vi "TP Information.vi"(10 "TP information in":string[](array[string]), 11 "base path":path) -> (2 "TP Information out":string[](array[string]))   [LabVIEW 2018]
uses:
  Global.vi
panel:
  out "布尔":bool
  in  "Bar":bool
  in  "过程停止按钮":bool
  in  "HW Ch Number":string caption="硬体配置通道数"
  in  "Board COL":string caption="连板方式(列)"
  in  "Board ROW":string caption="连板方式(行)"
  in  "确定":bool
  in  "浏览":bool
  in  "hwfile":string caption="配置文件"
  in  "备注":string
  in  "author":string caption="用户："
  in  "Modulename":string caption="机种名称"
  # "X"
  # "="
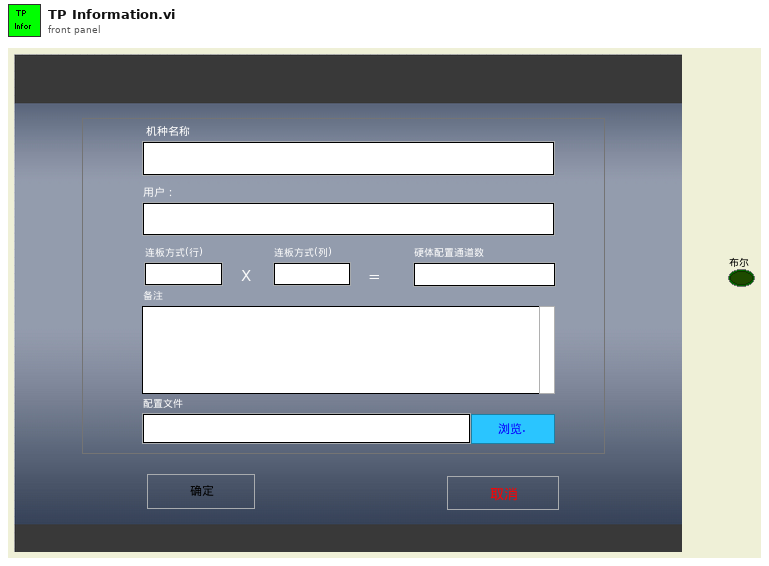
[diagram p1: front panel]
types:
  T1 = typedef "Window Refnum.ctl" = refnum<k1>
  T2 = typedef "Window Rectangle.ctl" = cluster{"left":i16, "top":i16, "right":i16, "bottom":i16}
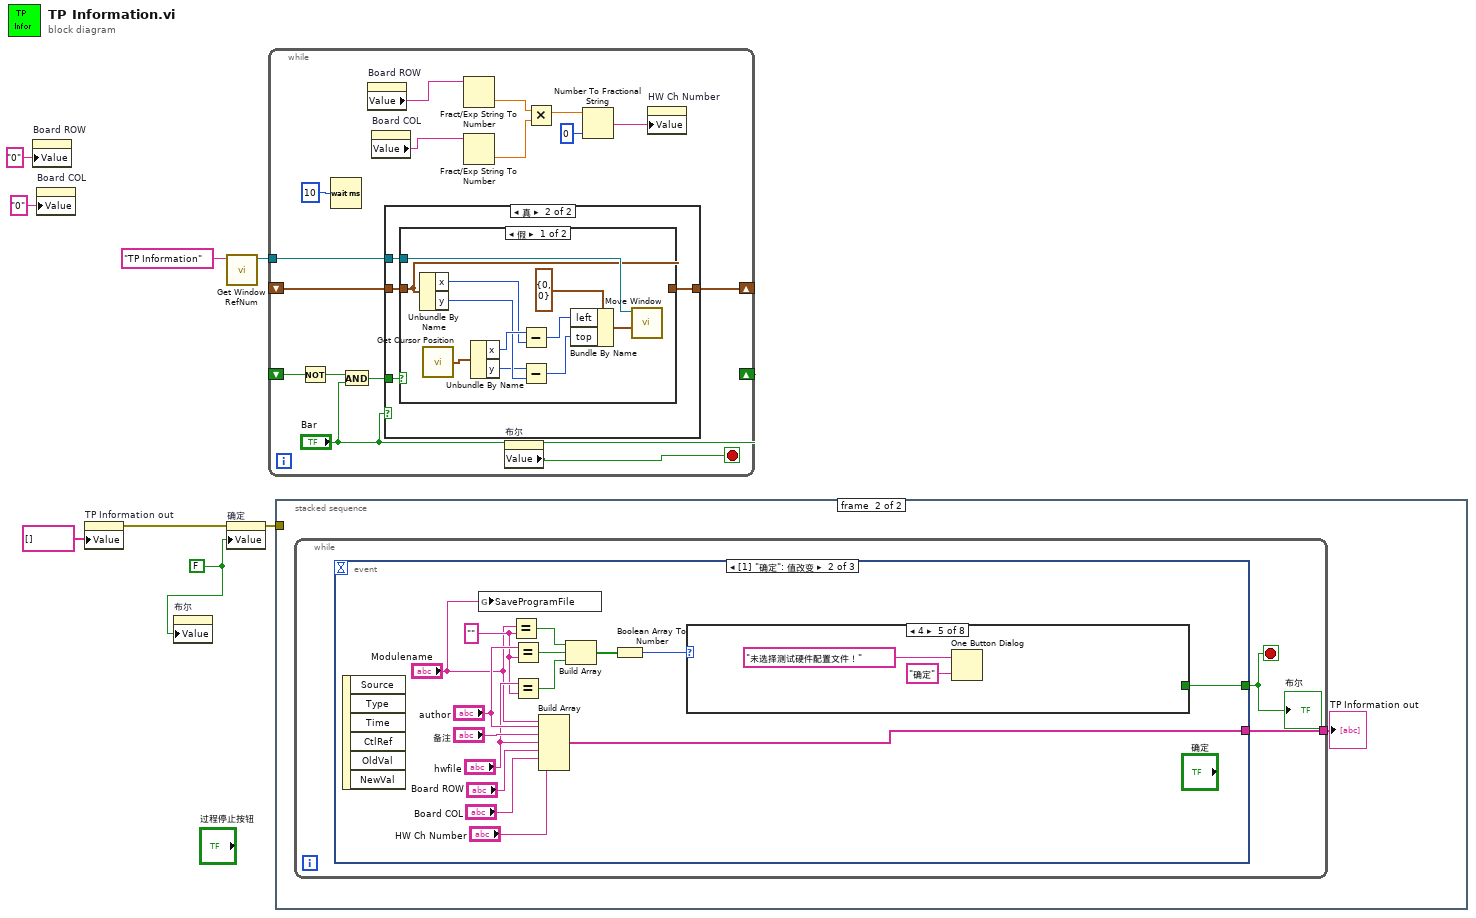
[diagram p0: block diagram]
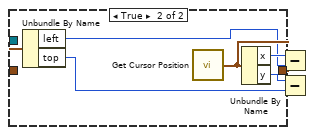
[diagram p3: hidden frame]
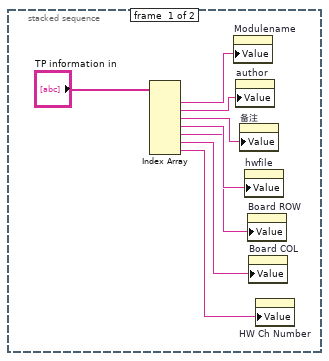
[diagram p4: hidden frame]
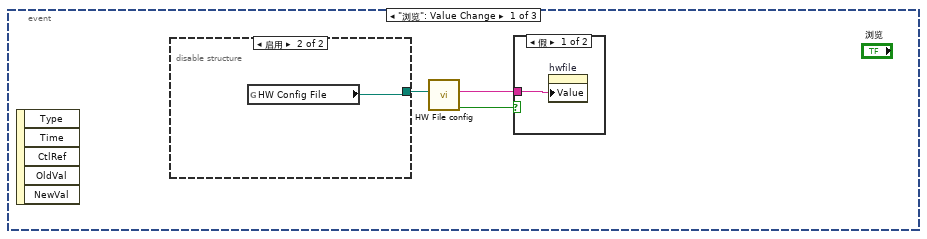
[diagram p5: hidden frame]
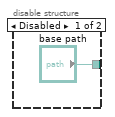
[diagram p6: hidden frame]
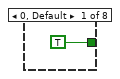
[diagram p8: hidden frame]
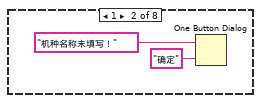
[diagram p9: hidden frame]
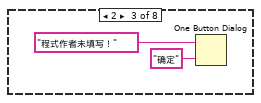
[diagram p10: hidden frame]
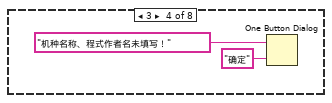
[diagram p11: hidden frame]
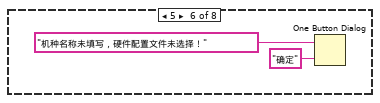
[diagram p12: hidden frame]
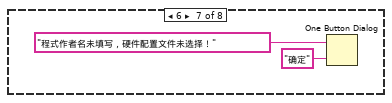
[diagram p13: hidden frame]
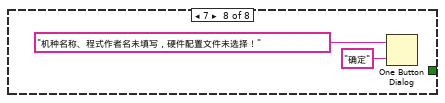
[diagram p14: hidden frame]
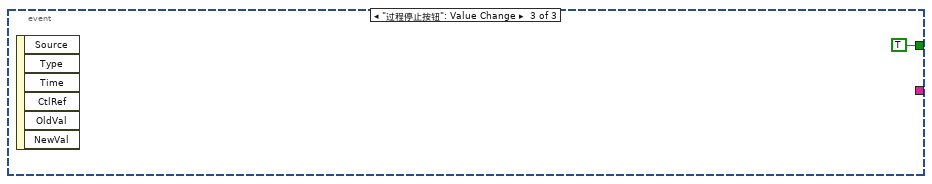
[diagram p15: hidden frame]
diagram:
  w3 = FALSE
  n1 = property on="Board ROW" class="Str"("Value"="0" ("Board ROW")) -> ()  [unwired: 2 in, 2 out]
  n2 = property on="Board COL" class="Str"("Value"="0" ("Board COL")) -> ()  [unwired: 2 in, 2 out]
  n3 = property on="TP Information out" class="Arr (严格)"("Value"=string[] []) -> (error out=w7:errorcluster)  [unwired: 2 in, 1 out]
  n4 = property on="布尔" class="Bool (严格)"("Value"=w3) -> ()  [unwired: 2 in, 2 out]
  n5 = call "Get Window RefNum.vi"("window name (\"\")"="TP Information" ("window name (\"\")")) -> ("window refnum (NaWR)"=w4:T1)  [unwired: 1 in, 7 out]
  n6 = property on="确定" class="Bool"(error in=w7, "Value"=w3) -> (error out=w8:errorcluster)  [unwired: 1 in, 1 out]
  n7 = while {
    shift-left: _ -> [w18]
    shift-right: [w19] -> _
    shift-left: _ -> [w22]
    shift-right: ["Bar"] -> _
    tunnel: w4 -> [w23]
    stop <- w16 stop-if-true
    n8 = Not(x=w22) -> (.not. x?=w21:bool)
    n9 = Wait (ms)(milliseconds to wait=u32 10) -> ()  [unwired: 1 out]
    n10 = And(x=w21, y="Bar") -> (x .and. y?=w17:bool)
    n11 = property on="Board ROW" class="Str"() -> ("Value"=w15:string)  [unwired: 2 in, 2 out]
    n12 = property on="Board COL" class="Str"() -> ("Value"=w14:string)  [unwired: 2 in, 2 out]
    n13 = case shown="真" "Bar" {
      tunnel: w23 -> [_ w29]
      tunnel: [w25 w28] -> w19
      tunnel: w18 -> [w25 w26]
      tunnel: w17 -> [_ w27]
      frame False {
      }
      frame True {
        n14 = case shown="假" w27 {
          tunnel: w29 -> [w35 w51]
          tunnel: [w30 w41] -> w28
          tunnel: w26 -> [w30 _]
          frame False {
            n15 = Unbundle By Name(w30) -> ("x"=w38:i16, "y"=w37:i16)
            n16 = call "Get Cursor Position.vi"() -> ("cursor position"=w40:cluster{"x":i16, "y":i16})
            n17 = Unbundle By Name(w40) -> ("x"=w39:i16, "y"=w36:i16)
            n18 = Subtract(x=w39, y=w38) -> (x-y=w32:i16)
            n19 = Subtract(x=w36, y=w37) -> (x-y=w33:i16)
            n20 = Bundle By Name(cluster=cluster{"left":i16, "top":i16} {"left"=0, "top"=0} ("new position (0,0)"), "left"=w32, "top"=w33) -> (w31:cluster{"left":i16, "top":i16})
            n21 = call "Move Window.vi"("new position (0,0)"=w31, "window refnum (NaWR)"=w35) -> ()  [unwired: 2 in, 4 out]
          }
          frame True {
            n22 = call "Get Window Rectangle.vi"("window refnum (NaWR)"=w51) -> ("window rect"=w50:T2)  [unwired: 1 in, 5 out]
            n23 = call "Extract Window Origin.vi"("window rect"=w50) -> ("window origin"=w49:cluster{"left":i16, "top":i16})  [unwired: 1 out]
            n24 = Unbundle By Name(w49) -> ("left"=w46:i16, "top"=w45:i16)
            n25 = call "Get Cursor Position.vi"() -> ("cursor position"=w48:cluster{"x":i16, "y":i16})
            n26 = Unbundle By Name(w48) -> ("x"=w47:i16, "y"=w44:i16)
            n27 = Subtract(x=w47, y=w46) -> (x-y=w42:i16)
            n28 = Subtract(x=w44, y=w45) -> (x-y=w43:i16)
            n29 = Bundle By Name(cluster=w48, "x"=w42, "y"=w43) -> (w41:cluster{"x":i16, "y":i16})
          }
        }
      }
    }
    n30 = Fract/Exp String To Number(string=w15) -> (number=w13:dbl)  [unwired: 3 in, 1 out]
    n31 = Fract/Exp String To Number(string=w14) -> (number=w12:dbl)  [unwired: 3 in, 1 out]
    n32 = property on="布尔" class="Bool (严格)"() -> ("Value"=w16:bool)  [unwired: 2 in, 2 out]
    n33 = Multiply(x=w13, y=w12) -> (x*y=w11:dbl)
    n34 = Number To Fractional String(number=w11, precision (6)=i16 0 ("精度(6)")) -> (F-format string=w9:string)  [unwired: 2 in]
    n35 = property on="HW Ch Number" class="Str"("Value"=w9) -> ()  [unwired: 2 in, 2 out]
  }
  n36 = stacked-sequence {
    tunnel: w8 -> [_ _]
    frame #0 {
      n37 = Index Array(array="TP information in") -> (element #1=w58:string, element #2=w57:string, element #3=w56:string, element #4=w55:string, element #5=w54:string, element #6=w53:string, element #7=w52:string)  [unwired: 7 in]
      n38 = property on="Modulename" class="Str"("Value"=w58) -> ()  [unwired: 2 in, 2 out]
      n39 = property on="author" class="Str"("Value"=w57) -> ()  [unwired: 2 in, 2 out]
      n40 = property on="备注" class="Str"("Value"=w56) -> ()  [unwired: 2 in, 2 out]
      n41 = property on="hwfile" class="Str"("Value"=w55) -> ()  [unwired: 2 in, 2 out]
      n42 = property on="Board ROW" class="Str"("Value"=w54) -> ()  [unwired: 2 in, 2 out]
      n43 = property on="Board COL" class="Str"("Value"=w53) -> ()  [unwired: 2 in, 2 out]
      n44 = property on="HW Ch Number" class="Str"("Value"=w52) -> ()  [unwired: 2 in, 2 out]
    }
    frame #1 {
      n45 = while {
        tunnel: [w61] -> w60
        stop <- w62 stop-if-true
        n46 = event shown="[1] \"确定\": 值改变" {
          selector: _ -> [_ _ _]
          dyn-events: _ -> [_ _ _]
          timeout: _ -> [_ _ _]
          tunnel: [_ w73 TRUE] -> w62
          tunnel: [_ w83 _] -> w61
          event "浏览": Value Change {
            n47 = event-data() -> ()  [unwired: 6 out]
            n48 = disable-structure shown="启用" {
              disable-tunnel: ["base path" w67] -> w65
              frame Disabled {
              }
              frame Enabled {
                n49 = global read "Global.vi" "HW Config File"() -> (w67:path)
              }
            }
            n50 = call "HW File config.vi"("base path"=w65) -> ("Cancel"=w64:bool, "count"=w63:string)  [unwired: 9 out]
            n51 = case shown="假" w64 {
              tunnel: w63 -> [w68 _]
              frame False {
                n52 = property on="hwfile" class="Str"("Value"=w68) -> ()  [unwired: 2 in, 2 out]
              }
              frame True {
              }
            }
          }
          event "确定": Value Change {
            w79 = ""
            n53 = event-data() -> ()  [unwired: 7 out]
            n54 = global write "Global.vi" "SaveProgramFile"("Modulename") -> ()
            n55 = Equal?(x="Modulename", y=w79) -> (x = y?=w78:bool)
            n56 = Equal?(x="author", y=w79) -> (x = y?=w77:bool)
            n57 = Equal?(x="hwfile", y=w79) -> (x = y?=w76:bool)
            n58 = Build Array("Modulename", "author", "备注", "hwfile", "Board ROW", "Board COL", "HW Ch Number") -> (w83:string[])
            n59 = Build Array(w78, w77, w76) -> (w75:bool[])
            n60 = Boolean Array To Number(Boolean array=w75) -> (number=w74:u32)
            n61 = case shown="4" w74 {
              tunnel: [TRUE _ _ _ _ _ _ _] -> w73
              frame 0, Default {
              }
              frame 1 {
                n62 = One Button Dialog(message="机种名称未填写！" ("消息"), button name ("OK")="确定" ("按钮名称（“确定”）")) -> ()  [unwired: 1 out]
              }
              frame 2 {
                n63 = One Button Dialog(message="程式作者未填写！" ("消息"), button name ("OK")="确定" ("按钮名称（“确定”）")) -> ()  [unwired: 1 out]
              }
              frame 3 {
                n64 = One Button Dialog(message="机种名称、程式作者名未填写！" ("消息"), button name ("OK")="确定" ("按钮名称（“确定”）")) -> ()  [unwired: 1 out]
              }
              frame 4 {
                n65 = One Button Dialog(message="未选择测试硬件配置文件！" ("消息"), button name ("OK")="确定" ("按钮名称（“确定”）")) -> ()  [unwired: 1 out]
              }
              frame 5 {
                n66 = One Button Dialog(message="机种名称未填写，硬件配置文件未选择！" ("消息"), button name ("OK")="确定" ("按钮名称（“确定”）")) -> ()  [unwired: 1 out]
              }
              frame 6 {
                n67 = One Button Dialog(message="程式作者名未填写，硬件配置文件未选择！" ("消息"), button name ("OK")="确定" ("按钮名称（“确定”）")) -> ()  [unwired: 1 out]
              }
              frame 7 {
                n68 = One Button Dialog(message="机种名称、程式作者名未填写，硬件配置文件未选择！" ("消息"), button name ("OK")="确定" ("按钮名称（“确定”）")) -> ()  [unwired: 1 out]
              }
            }
          }
          event "过程停止按钮": Value Change {
            n69 = event-data() -> ()  [unwired: 7 out]
          }
        }
        "布尔" <- w62
      }
      "TP Information out" <- w60
    }
  }
